vi "Calibrate NART DUT Example.vi"(3 "RFSA Handle In":T2="RIO0 (9)", 4 "OTP":bool, 5 "Max Input Power, dBm":T4=20.0 format="%.1f", 6 "Trigger":T7={"Source"=enum."Power", "Edge"=enum."Rising", "Delay, sec"=0.0, "Level, dBm"=-10.0, "Min Quiet Time, sec"=1.5e-05} {"Min Quiet Time, sec" format="%^.2e"; "Level, dBm" format="%.1f"; "Delay, sec" format="%^.2e"}, 7 "Calibration Data":T1 {"Calibration Table" min=0.0 max=127.0 format="%.2p"; "Time Stamp, sec" format="%^.2e"; "Temperature, C" format="%.1f"}, 8 "error in (no error)":errorcluster, 10 "Frequency and Tx Gain":T3[](array[typedef])=[{"Frequency"=2412, "TX Gain"=75, "LL"=62, "UL"=62}, {"Frequency"=5180, "TX Gain"=65, "LL"=62, "UL"=62}, {"Frequency"=5700, "TX Gain"=80, "LL"=62, "UL"=62}], 11 "CART TCP Connection In":refnum<k5>) -> (0 "error out":errorcluster, 2 "CART TCP Connection Out":refnum<k5>)   [LabVIEW 2011]
uses:
  <userlib>/niRF/niSystem/SA/Includes/niSYS - SA - INC - STYP - Trigger.ctl
  <userlib>/niRF/niSystem/SA/Includes/niSYS - SA - INC - STYP - Trigger Delay.ctl
  <userlib>/niRF/niSystem/SA/Includes/niSYS - SA - INC - STYP - Timeout.ctl
  <userlib>/niRF/niSystem/SA/Includes/niSYS - SA - INC - STYP - Frequency Reference.ctl
  <userlib>/niRF/niSystem/SA/Includes/niSYS - SA - INC - STYP - Max Input Power.ctl
  LVx Folder/Support/TypeDef/TX Cal Data Rate.ctl
  <userlib>/niRF/niSystem/SA/Includes/niSYS - RFSA - INC - STYP - Handle.ctl
  <userlib>/niRF/niSystem/SA/Includes/niSYS - SA - INC - STYP - RBW Filter.ctl
  <userlib>/niRF/niBasic/SA/Waveform/Includes/niBASIC - SA - Waveform - INC - STYP - Averaging.ctl
panel:
  out "time, ms":u32=1968
  in  "port":u16=3363
  in  "Frequency Reference":T5={" Reference Source"=enum."On Board Clock", "Frequency, Hz"=10000000.0, "Backplane Source"=enum."None"} {"Frequency, Hz" format="%^.6e"}
  in  "Timeout, sec":T6=10.0 format="%.3f"
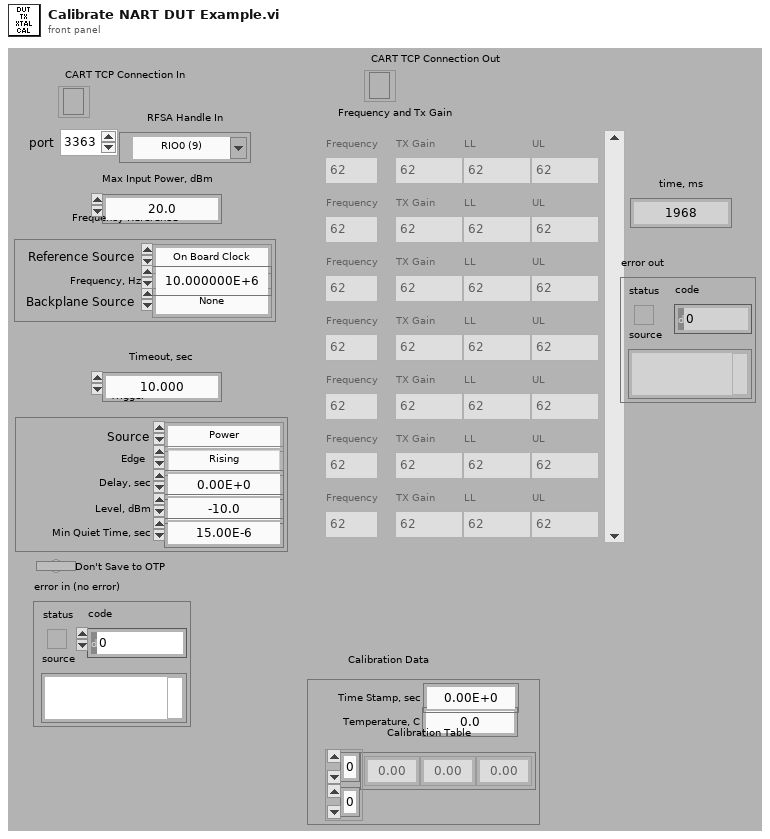
[diagram p1: front panel]
types:
  T1 = cluster{"Temperature, C":dbl, "Time Stamp, sec":dbl, "Calibration Table":dbl[][]}
  T2 = typedef "niSYS - RFSA - INC - STYP - Handle.ctl" = refnum<k15>
  T3 = typedef "TX Cal Data Rate.ctl" = cluster{"Frequency":u32, "TX Gain":u32, "LL":i32, "UL":u32}
  T4 = typedef "niSYS - SA - INC - STYP - Max Input Power.ctl" = dbl
  T5 = typedef "niSYS - SA - INC - STYP - Frequency Reference.ctl" = cluster{" Reference Source":enum16{"On Board Clock", "Ref In", "PXI Clock 10"}, "Frequency, Hz":dbl, "Backplane Source":enum16{"None", "Ref In", "On Board Clock"}}
  T6 = typedef "niSYS - SA - INC - STYP - Timeout.ctl" = dbl
  T7 = typedef "niSYS - SA - INC - STYP - Trigger.ctl" = cluster{"Source":enum16{"Immediate", "External", "Software", "RTSI 0", "RTSI 1", "RTSI 2", "RTSI 3", "RTSI 4", "RTSI 5", "RTSI 6", "RTSI 7", "PFI 0", "PFI 1", "PFI 2", "PXI Star", "Power"}, "Edge":enum16{"Rising", "Falling"}, "Delay, sec":T8, "Level, dBm":dbl, "Min Quiet Time, sec":dbl}
  T8 = typedef "niSYS - SA - INC - STYP - Trigger Delay.ctl" = dbl
  T9 = typedef "niBASIC - SA - Waveform - INC - STYP - Averaging.ctl" = cluster{"Averages":i32, "Average State":enum16{"Off", "On"}, "Average Mode":enum16{"Exponential", "Repeat"}, "Average Type":enum16{"RMS", "Log", "Scalar", "Max", "Min"}}
  T10 = typedef "niSYS - SA - INC - STYP - RBW Filter.ctl" = cluster{"Type":enum16{"Gaussian", "Flat", "None"}, "Bandwidth, Hz":dbl}
  T11 = typedef "niBASIC - SA - Waveform - INC - STYP - Measurement Handle.ctl" = refnum<notifier>
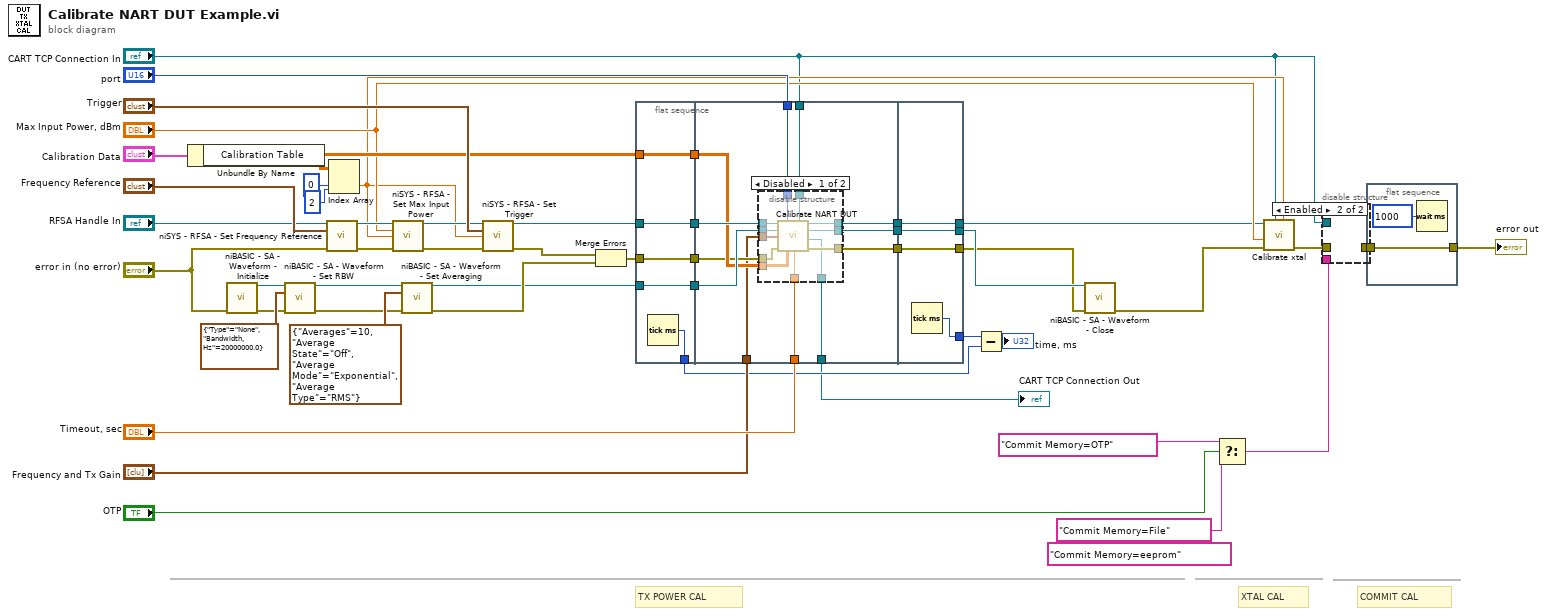
[diagram p0: block diagram]
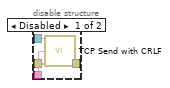
[diagram p2: hidden frame]
diagram:
  (unwired) "Commit Memory=eeprom"
  # "COMMIT CAL"
  # "XTAL CAL"
  # "TX POWER CAL"
  n1 = Unbundle By Name("Calibration Data") -> ("Calibration Table"=w14:dbl[][])
  n2 = call <userlib>:"niBASIC - SA - Waveform - Initialize.vi"("error in (no error)"="error in (no error)") -> ("Measurement Handle Out"=w46:T11, "error out"=w45:errorcluster)  [unwired: 1 in, 12 out]
  n3 = call <userlib>:"niBASIC - SA - Waveform - Set RBW.vi"("Measurement Handle In"=w46, "Resolution Bandwidth Filter"=T10 {"Type"=enum."None", "Bandwidth, Hz"=20000000.0} ("RBW Filter"), "error in (no error)"=w45) -> ("Measurement Handle Out"=w37:T11, "error out"=w36:errorcluster)  [unwired: 11 out]
  n4 = call <userlib>:"niSYS - RFSA - Set Frequency Reference.vi"("RFSA Handle In"="RFSA Handle In", "Frequency Reference"="Frequency Reference", "error in (no error)"="error in (no error)") -> ("RFSA Handle Out"=w48:T2, "error out"=w47:errorcluster)  [unwired: 1 in, 10 out]
  n5 = Index Array(array=w14, index (row)=0 ("disabled index (row)"), index (col)=2 ("disabled index (col)")) -> (element=w6:dbl)
  n6 = call <userlib>:"niSYS - RFSA - Set Max Input Power.vi"("RFSA Handle In"=w48, "Max Input Power, dBm"="Max Input Power, dBm", "External Attenuation, dB"=w6, "error in (no error)"=w47) -> ("RFSA Handle Out"=w34:T2, "error out"=w33:errorcluster)  [unwired: 10 out]
  n7 = call <userlib>:"niBASIC - SA - Waveform - Set Averaging.vi"("Measurement Handle In"=w37, "Averaging"=T9 {"Averages"=10, "Average State"=enum."Off", "Average Mode"=enum."Exponential", "Average Type"=enum."RMS"} ("Waveform Averaging"), "error in (no error)"=w36) -> ("Measurement Handle Out"=w40:T11, "error out"=w43:errorcluster)  [unwired: 11 out]
  n8 = call <userlib>:"niSYS - RFSA - Set Trigger.vi"("RFSA Handle In"=w34, "Trigger"="Trigger", "External Attenuation, dB"=w6, "error in (no error)"=w33) -> ("RFSA Handle Out"=w41:T2, "error out"=w44:errorcluster)  [unwired: 10 out]
  n9 = Merge Errors(w44, w43) -> (w38:errorcluster)
  n10 = flat-sequence {
    tunnel: w38 -> [w53]
    tunnel: w14 -> [w54]
    tunnel: w40 -> [w55]
    tunnel: w41 -> [w56]
    tunnel: [w56] -> w28
    tunnel: [w55] -> w27
    tunnel: [w54] -> w26
    tunnel: [w53] -> w25
    tunnel: [w52] -> w23
    tunnel: "Timeout, sec" -> [w62]
    tunnel: "Frequency and Tx Gain" -> [w60]
    tunnel: "port" -> [w59]
    tunnel: [w66] -> w31
    tunnel: [w65] -> w30
    tunnel: [w64] -> w29
    tunnel: w28 -> [w68]
    tunnel: w27 -> [w67]
    tunnel: w26 -> [w63]
    tunnel: w25 -> [w61]
    tunnel: "CART TCP Connection In" -> [w58]
    tunnel: [w57] -> w20
    tunnel: [w82] -> w8
    tunnel: [w83] -> w19
    tunnel: [w84] -> w7
    tunnel: w31 -> [w84]
    tunnel: w30 -> [w83]
    tunnel: w29 -> [w82]
    tunnel: [w81] -> w24
    frame #0 {
      n11 = Tick Count (ms)() -> (millisecond timer value=w52:u32)
    }
    frame #1 {
      n12 = disable-structure shown="Disabled" {
        disable-tunnel: w68 -> [w80 _]
        disable-tunnel: w67 -> [w79 _]
        disable-tunnel: [w78 _] -> w66
        disable-tunnel: [w77 _] -> w65
        disable-tunnel: [w76 _] -> w64
        disable-tunnel: w63 -> [w75 _]
        disable-tunnel: w62 -> [w74 _]
        disable-tunnel: w61 -> [w73 _]
        disable-tunnel: w60 -> [w72 _]
        disable-tunnel: w59 -> [w71 _]
        disable-tunnel: w58 -> [w70 _]
        disable-tunnel: [w69 _] -> w57
        frame Disabled {
          n13 = call "Calibrate NART DUT.vi"("RFSA Device"=w80, "port"=w71, "CART TCP Connection In"=w70, "Measurement Handle In"=w79, "Frequency and Tx Gain"=w72, "error in (no error)"=w73, "Path Loss, dB"=w75, "Measurement Timeout, sec"=w74) -> ("RFSA Handle Out"=w78:T2, "Measurement Handle Out"=w77:T11, "CART TCP Connection Out"=w69:refnum<k5>, "error out"=w76:errorcluster)  [unwired: 4 in]
        }
        frame Enabled {
        }
      }
    }
    frame #2 {
      n14 = Tick Count (ms)() -> (millisecond timer value=w81:u32)
    }
  }
  n15 = Subtract(x=w24, y=w23) -> (x-y=→"time, ms":u32)
  n16 = call <userlib>:"niBASIC - SA - Waveform - Close.vi"("Measurement Handle In"=w19, "error in (no error)"=w8) -> ("error out"=w9:errorcluster)  [unwired: 13 out]
  n17 = Select(t="Commit Memory=OTP", s="OTP", f="Commit Memory=File") -> (s? t:f=w1:string)
  n18 = call "Calibrate xtal.vi"("External Attenuation, dB"=w6, "CART TCP Connection In"="CART TCP Connection In", "Error In"=w9, "Max Input Power, dBm"="Max Input Power, dBm", "RFSA Device"=w7) -> ("error out"=w5:errorcluster)  [unwired: 6 in]
  n19 = disable-structure shown="Enabled" {
    disable-tunnel: w5 -> [w88 _]
    disable-tunnel: "CART TCP Connection In" -> [w87 _]
    disable-tunnel: [w86 _] -> w3
    disable-tunnel: w1 -> [w85 _]
    frame Disabled {
      n20 = call "TCP Send with CRLF.vi"("CART TCP Connection"=w87, "data in"=w85, "error IO"=w88) -> ("error out"=w86:errorcluster)  [unwired: 11 in, 1 out]
    }
    frame Enabled {
    }
  }
  n21 = flat-sequence {
    tunnel: w3 -> [w90]
    tunnel: [w90] -> w2
    frame #0 {
      n22 = Wait (ms)(milliseconds to wait=u32 1000) -> ()  [unwired: 1 out]
    }
  }
  "error out" <- w2
  "CART TCP Connection Out" <- w20
